vi "Compute Max Level.vi"(0 "ToneCloud in":refnum<class "Tone Cloud.lvclass">, 1 "Filter in":refnum<class "Filter.lvclass">, 5 "Level in":refnum<class "Level.lvclass">, 7 "Fs (Hz)":dbl, 9 "Vmax":dbl, 11 "error in (no error)":errorcluster) -> (4 "ToneCloud out":refnum<class "Tone Cloud.lvclass">, 6 "Level thru":refnum<class "Level.lvclass">, 10 "Lmax":dbl, 15 "error out":errorcluster)   [LabVIEW 2020, in "Tone Cloud.lvclass"]
uses:
  Tone Cloud.lvclass
  Level/Level.lvclass
  Filter/Filter.lvclass
  Tone Cloud.lvclass/Tone Cloud.ctl
  5383cbb3-07a5-4200-b90b-401089faa7f7.vi
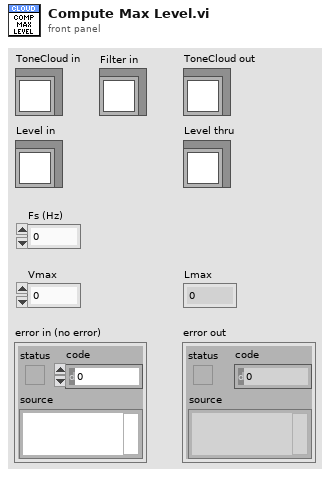
[diagram p1: front panel]
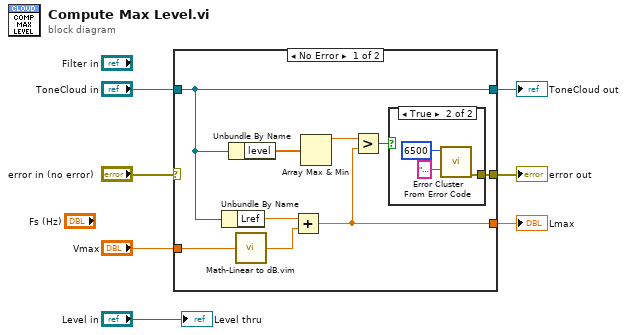
[diagram p0: block diagram]
diagram:
  n1 = case shown="No Error" "error in (no error)" {
    selector: "error in (no error)" -> [_ w20]
    tunnel: [w16 w21] -> w6
    tunnel: "ToneCloud in" -> [w16 w21]
    tunnel: "Vmax" -> [w11 _]
    tunnel: [w8 _] -> w2
    tunnel: [w12 w20] -> w1
    frame No Error {
      n2 = Unbundle By Name(w16) -> ("Lref"=w10:dbl)
      n3 = Unbundle By Name(w16) -> ("level"=w15:dbl[])
      n4 = call "Math-Linear to dB.vim"("linear"=w11) -> ("dB"=w9:dbl)
      n5 = Add(x=w10, y=w9) -> (x+y=w8:dbl)
      n6 = Array Max & Min(array=w15) -> (max value=w14:dbl)  [unwired: 3 out]
      n7 = Greater?(x=w14, y=w8) -> (0:w13:bool)
      n8 = case shown="True" w13 {
        tunnel: [_ w17] -> w12
        frame False {
        }
        frame True {
          n9 = call <vilib>:"Error Cluster From Error Code.vi"("error message (\"\")"="Tone cloud max level is likely unachievable." ("error message (\"\")"), "error code (0)"=6500) -> ("error out"=w17:errorcluster)  [unwired: 7 in]
        }
      }
    }
    frame Error {
    }
  }
  "error out" <- w1
  "ToneCloud out" <- w6
  "Lmax" <- w2
  "Level thru" <- "Level in"
